vi "Speed data viewer.vi"() -> ()   [LabVIEW 2020]
uses:
  <userlib>/My Palettes.lib/Files & paths/Spreadsheet/Read From Spreadsheet File (string)-Mod.vi
  User Interface/Visualisation/Timelapse Viewer/Globals/gl_Time series viewer globals.vi
  User Interface/Visualisation/Timelapse Viewer/Typedefs/Time series viewer refs.ctl
panel:
  in  "Speed data file":path
  out "error out":errorcluster
  out "Error":bool
  in  "Trial number":i32=1 min=0 max=0 step=1
  in  "Mode":enum16{"All trials", "Single trial"}(ring)
  out "Valid speed data array":dbl[](graph) caption="SPEED DATA GRAPH"
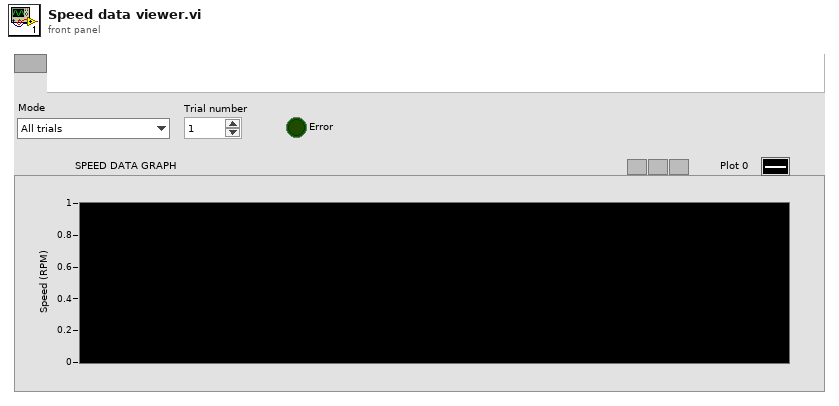
[diagram p1: front panel]
types:
  T1 = typedef "Time series viewer refs.ctl" = cluster{"This VI":refnum<vi>, "Image control":refnum<vi>, "AVI Mode ind":refnum<vi>, "Play":refnum<vi>, "Stop":refnum<vi>, "Back":refnum<vi>, "Scrollbar":refnum<vi>, "Video length info":refnum<vi>, "Expected speed values":refnum<vi>, "Intensity":refnum<vi>, "Path":refnum<vi>, "Selection sliders":refnum<vi>, "Speed Graph ref":refnum<vi>, "Frame rate set (fps)":refnum<vi>, "Number of rows to generate":refnum<vi>, "VL Image Array":refnum<vi>, "Image Scrollbar":refnum<vi>, "Channel to load":refnum<vi>, "Colour":refnum<vi>}
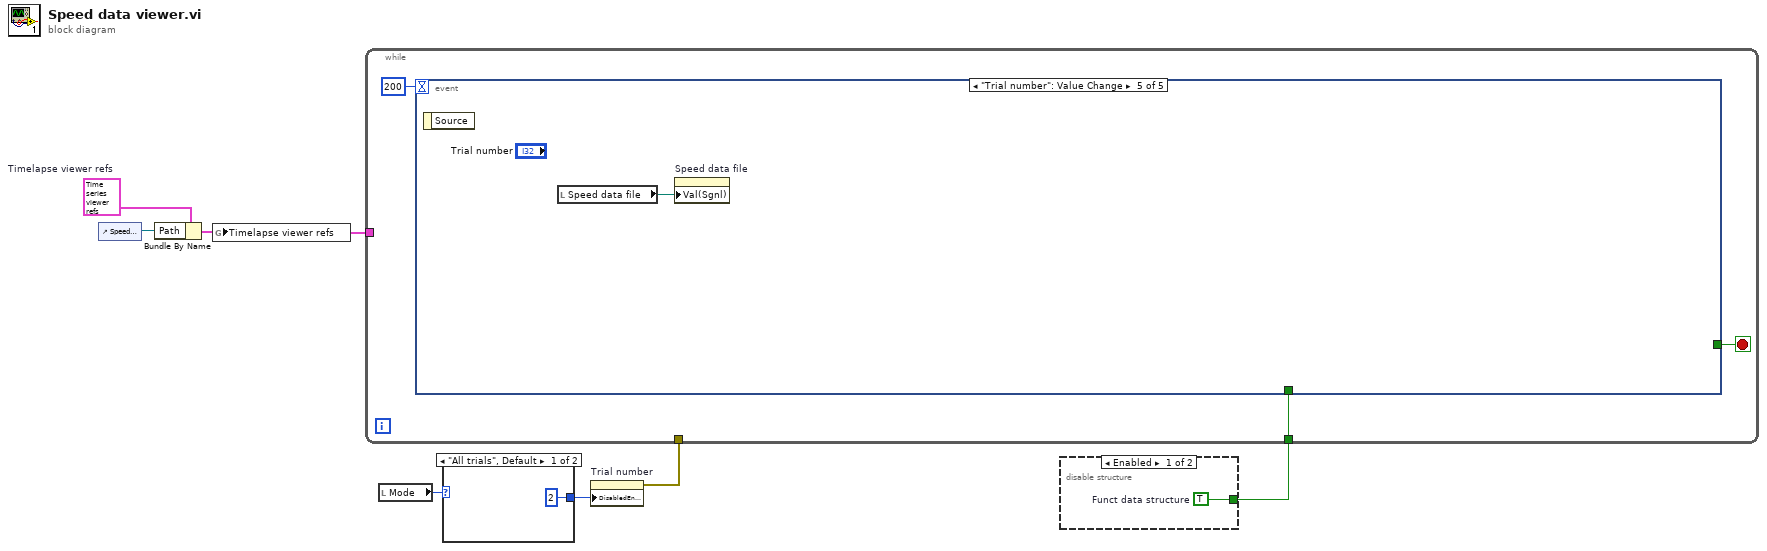
[diagram p0: block diagram]
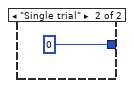
[diagram p3: hidden frame]
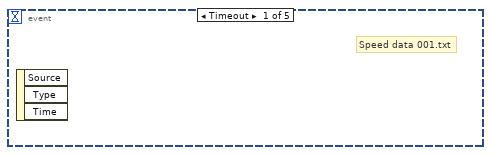
[diagram p4: hidden frame]
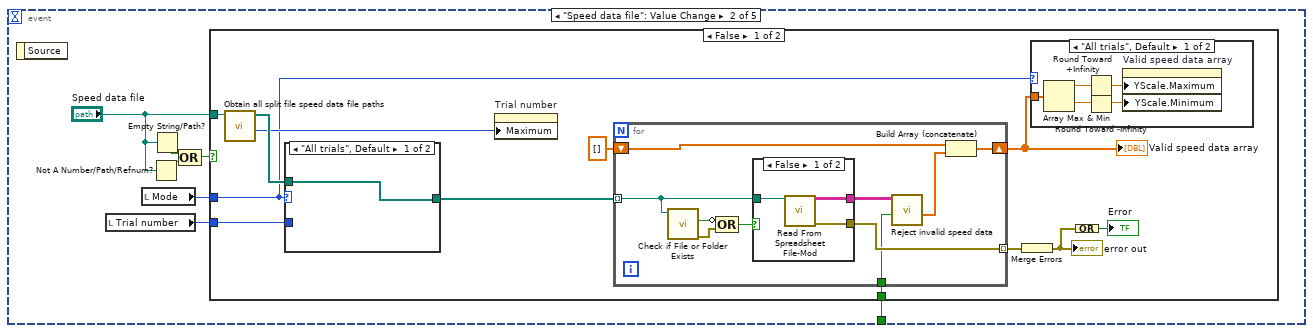
[diagram p5: hidden frame]
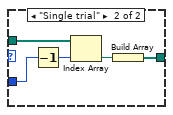
[diagram p8: hidden frame]
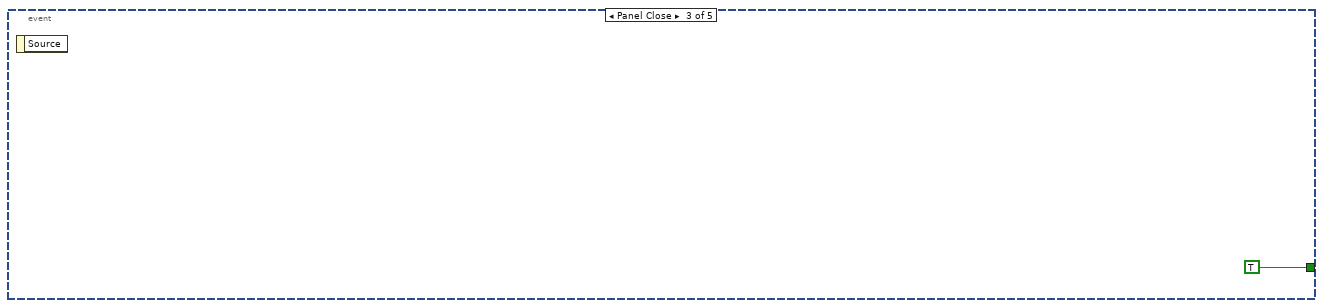
[diagram p10: hidden frame]
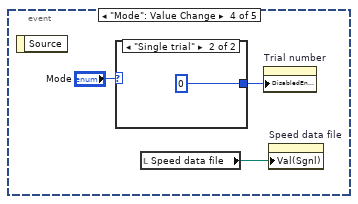
[diagram p11: hidden frame]
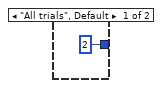
[diagram p12: hidden frame]
diagram:
  w3 = T1 {"This VI"=refnum, "Image control"=refnum, "AVI Mode ind"=refnum, "Play"=refnum, "Stop"=refnum, "Back"=refnum, "Scrollbar"=refnum, "Video length info"=refnum, "Expected speed values"=refnum, "Intensity"=refnum, "Path"=refnum, "Selection sliders"=refnum, "Speed Graph ref"=refnum, "Frame rate set (fps)"=refnum, "Number of rows to generate"=refnum, "VL Image Array"=refnum, "Image Scrollbar"=refnum, "Channel to load"=refnum, "Colour"=refnum}  # Timelapse viewer refs
  n1 = control-ref of="Speed data file"() -> (w1:refnum<vi>)
  n2 = Bundle By Name(cluster=w3, "Path"=w1) -> (w2:T1)
  n3 = global write "gl_Time series viewer globals.vi" "Timelapse viewer refs"(w2) -> ()
  n4 = local read "Mode"() -> (w5:enum16{"All trials", "Single trial"})
  n5 = case shown="\"All trials\", Default" w5 {
    tunnel: [2 0] -> w7
    frame "All trials", Default {
    }
    frame "Single trial" {
    }
  }
  n6 = property on="Trial number" class="DigNum (strict)"("DisabledEnum"=w7) -> (error out=w6:errorcluster)  [unwired: 2 in, 1 out]
  n7 = disable-structure shown="Enabled" {
    disable-tunnel: [w10 _] -> w4
    frame Enabled {
      w10 = TRUE  # Funct data structure
    }
    frame Disabled {
    }
  }
  n8 = while {
    tunnel: w6 -> [_]
    tunnel: w4 -> [w11]
    tunnel: w2 -> [_]
    stop <- w12 stop-if-true
    n9 = event shown="[4] \"Trial number\": Value Change" {
      selector: _ -> [_ _ _ _ _]
      dyn-events: _ -> [_ _ _ _ _]
      timeout: 200 -> [_ _ _ _ _]
      tunnel: [_ _ TRUE _ _] -> w12
      tunnel: w11 -> [_ w15 _ _ _]
      event Timeout {
        # "Speed data 001.txt"
        n10 = event-data() -> ()  [unwired: 1 in, 3 out]
      }
      event "Speed data file": Value Change {
        n11 = event-data() -> ()  [unwired: 1 in, 1 out]
        n12 = local read "Trial number"() -> (w16:i32)
        n13 = local read "Mode"() -> (w17:enum16{"All trials", "Single trial"})
        n14 = Not A Number/Path/Refnum?(number/path/refnum="Speed data file") -> (NaN/Path/Refnum?=w19:bool)
        n15 = Empty String/Path?(string/path="Speed data file") -> (empty?=w20:bool)
        n16 = Compound Arithmetic op=OR(w20, w19) -> (w18:bool)
        n17 = case shown="False" w18 {
          tunnel: "Speed data file" -> [w32 _]
          tunnel: w17 -> [w24 _]
          tunnel: w16 -> [w29 _]
          tunnel: w15 -> [w21 _]
          frame False {
            n18 = call "Obtain all split file speed data file paths.vi"("Speed data file path & name (any)"=w32) -> ("Number of speed data split files (= number of trials)"=w30:i32, "Trial speed data split file paths"=w31:path[])  [unwired: 9 in]
            n19 = case shown="\"All trials\", Default" w24 {
              tunnel: w31 -> [w51 w56]
              tunnel: w29 -> [_ w54]
              tunnel: [w51 w52] -> w28
              frame "All trials", Default {
              }
              frame "Single trial" {
                n20 = Decrement(x=w54) -> (x-1=w55:i32)
                n21 = Index Array(array=w56, index=w55) -> (element=w53:path)
                n22 = Build Array(w53) -> (w52:path[])
              }
            }
            n23 = property on="Trial number" class="DigNum (strict)"("Maximum"=w30) -> ()  [unwired: 2 in, 2 out]
            n24 = for {
              tunnel: w28 -> [w43] mode=indexing
              shift-right: [w41] -> w26
              shift-left: dbl[] [] -> [w40]
              tunnel: [w39] -> w25 mode=indexing
              tunnel: w21 -> [w38]
              n25 = call <vilib>:"Check if File or Folder Exists.vi"("path"=w43) -> ("error out"=w45:errorcluster, "file or folder exists?"=w46:bool)  [unwired: 8 in, 1 out]
              n26 = Compound Arithmetic op=OR(invert w46, w45) -> (w47:bool)
              n27 = case shown="False" w47 {
                tunnel: w43 -> [w50 _]
                tunnel: [w49 _] -> w44
                tunnel: [w48 _] -> w39
                frame False {
                  n28 = call-poly <userlib>:"Read From Spreadsheet File-Mod.vi"("file path (dialog if empty)"=w50) -> ("all rows"=w49:string[][], "error out"=w48:errorcluster)  [unwired: 9 in, 4 out]
                }
                frame True {
                }
              }
              n29 = call "Reject invalid speed data.vi"("Funct data structure"=w38, "Spreadsheet data"=w44) -> ("Valid speed data"=w42:dbl[])  [unwired: 7 in, 2 out]
              n30 = Build Array (concatenate)(w40, w42) -> (w41:dbl[])
            }
            "Valid speed data array" <- w26
            n31 = Merge Errors(w25) -> (w23:errorcluster)
            "error out" <- w23
            n32 = case shown="\"All trials\", Default" w24 {
              tunnel: w26 -> [w33 _]
              frame "All trials", Default {
                n33 = Array Max & Min(array=w33) -> (max value=w35:dbl, min value=w34:dbl)  [unwired: 2 out]
                n34 = Round Toward +Infinity(x=w35) -> (ceil(x): smallest int >= x=w36:dbl)
                n35 = Round Toward -Infinity(1:w34) -> (0:w37:dbl)
                n36 = property on="Valid speed data array" class="WFGraph (strict)"("YScale.Maximum"=w36, "YScale.Minimum"=w37) -> ()  [unwired: 2 in, 2 out]
              }
              frame "Single trial" {
              }
            }
            n37 = Compound Arithmetic op=OR(w23) -> (→"Error":bool)
          }
          frame True {
          }
        }
      }
      event Panel Close {
        n38 = event-data() -> ()  [unwired: 1 in, 1 out]
      }
      event "Mode": Value Change {
        n39 = event-data() -> ()  [unwired: 1 in, 1 out]
        n40 = case shown="\"Single trial\"" "Mode" {
          tunnel: [2 0] -> w58
          frame "All trials", Default {
          }
          frame "Single trial" {
          }
        }
        n41 = local read "Speed data file"() -> (w60:path)
        n42 = property on="Trial number" class="DigNum (strict)"("DisabledEnum"=w58) -> ()  [unwired: 2 in, 2 out]
        n43 = property on="Speed data file" class="Path"("Val(Sgnl)"=w60) -> ()  [unwired: 2 in, 2 out]
      }
      event "Trial number": Value Change {
        n44 = event-data() -> ()  [unwired: 1 in, 1 out]
        n45 = local read "Speed data file"() -> (w63:path)
        n46 = property on="Speed data file" class="Path"("Val(Sgnl)"=w63) -> ()  [unwired: 2 in, 2 out]
      }
    }
  }
